vi "SendCommand.vi"(8 "error in (no error)":errorcluster, 10 "Data in":variant, 11 "Commands":T1) -> (0 "error out":errorcluster)   [LabVIEW 2015]
uses:
  TypeDef/RequestHandlerCommands.ctl
  TypeDef/RequestHandlerQueueCluster.ctl
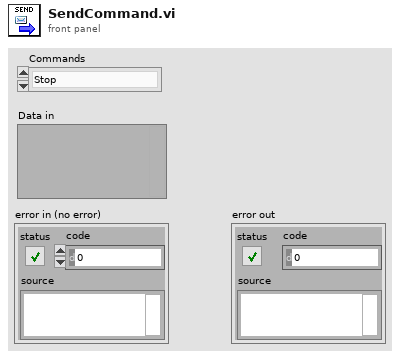
[diagram p1: front panel]
types:
  T1 = typedef "RequestHandlerCommands.ctl" = enum16{"Stop", "IntoRoom", "OutOfRoom"}
  T2 = typedef "RequestHandlerQueueCluster.ctl" = cluster{"Commands":T1, "Data":variant}
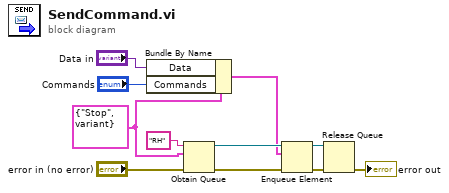
[diagram p0: block diagram]
diagram:
  w9 = T2 {"Commands"=enum."Stop", "Data"=variant} ("Queue Cluster")
  n1 = Bundle By Name(cluster=w9, "Data"="Data in", "Commands"="Commands") -> (w1:T2)
  n2 = Obtain Queue(name (unnamed)="RH", element data type=w9, error in (no error)="error in (no error)") -> (queue out=w5:refnum<queue>, error out=w7:errorcluster)  [unwired: 2 in, 1 out]
  n3 = Enqueue Element(queue=w5, element=w1, error in (no error)=w7) -> (queue out=w6:refnum<queue>, error out=w8:errorcluster)  [unwired: 1 in, 1 out]
  n4 = Release Queue(queue=w6, error in (no error)=w8) -> (error out=→"error out":errorcluster)  [unwired: 1 in, 2 out]
